vi "Add Controls in Configuration.vi"(0 "new code module":path, 1 "vi reference":refnum<vi>, 2 "configuration ctl refnum":refnum<vi>, 11 "error in":errorcluster) -> (4 "controls reference":refnum<vi>[](array[refnum]), 15 "error out":errorcluster)   [LabVIEW 2021, in "Converter.lvlib"]
uses:
  Converter.lvlib
  Converter Reusables/Converter Reusables.lvlib
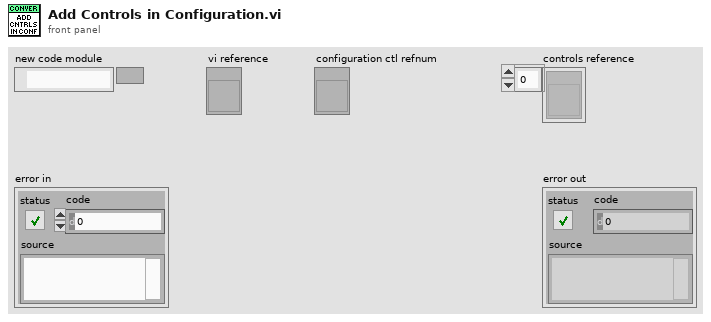
[diagram p1: front panel]
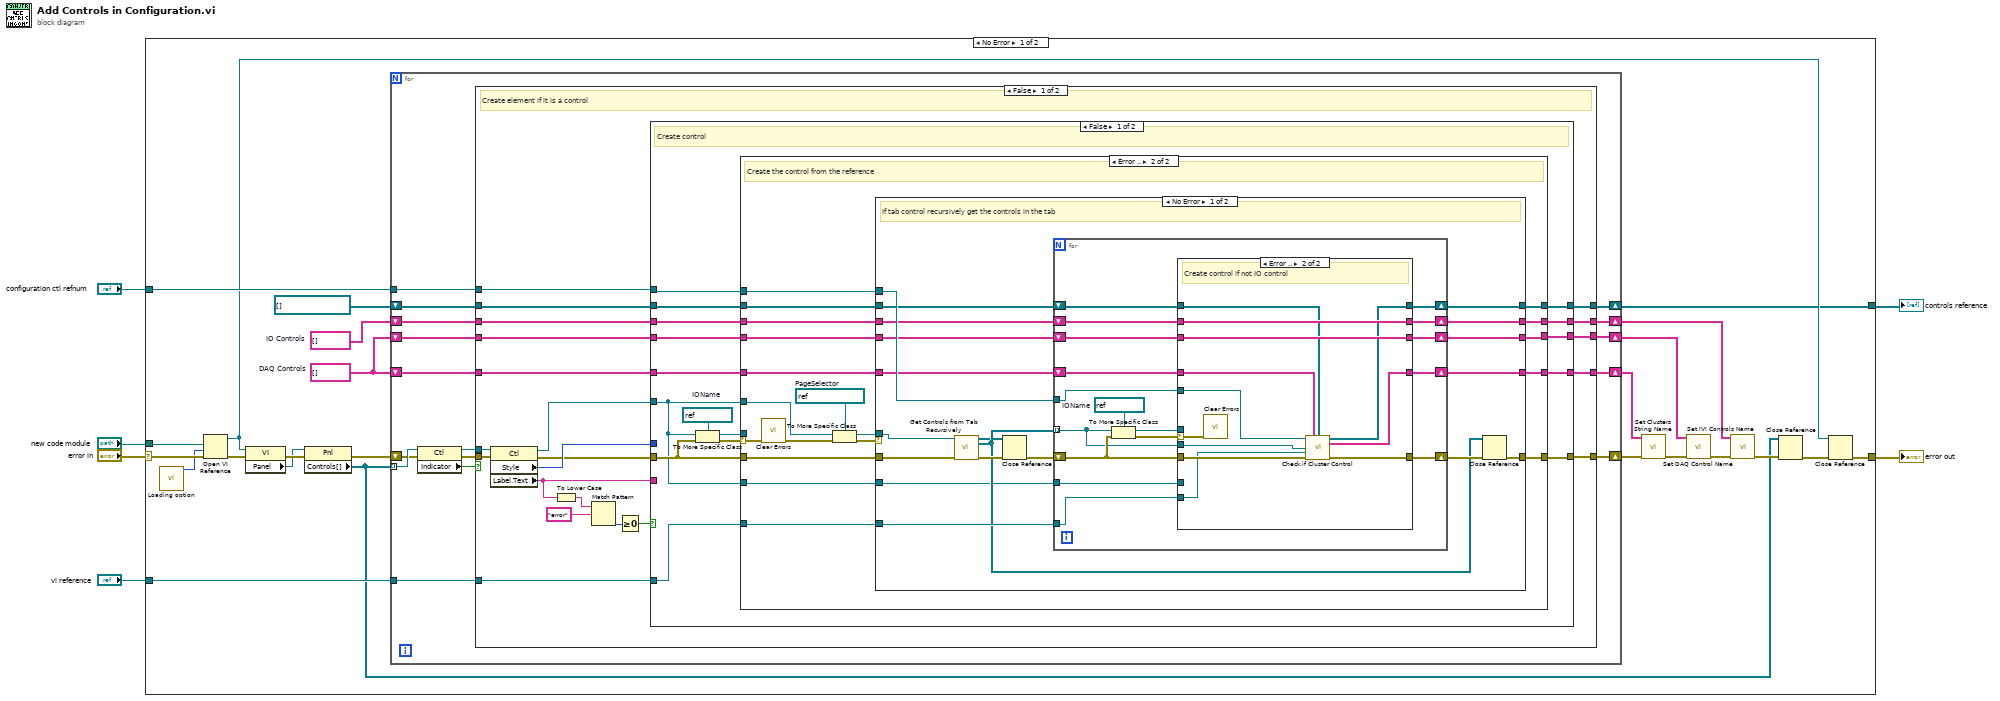
[diagram p0: block diagram]
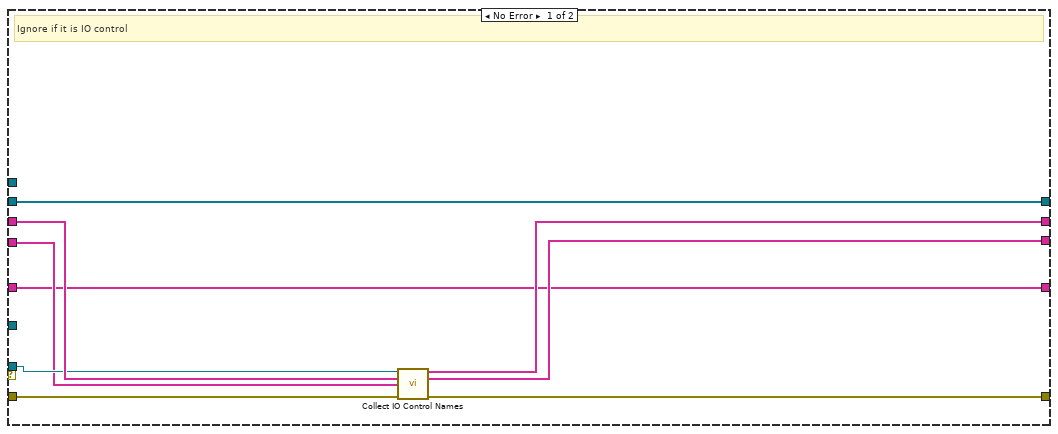
[diagram p2: hidden frame]
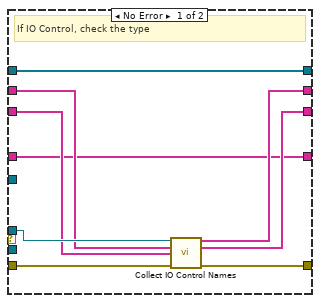
[diagram p3: hidden frame]
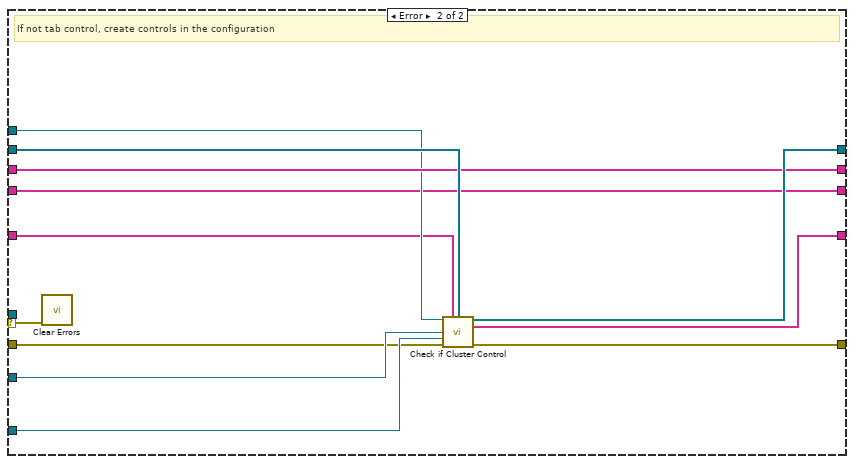
[diagram p4: hidden frame]
diagram:
  n1 = case shown="No Error" "error in" {
    selector: "error in" -> [w8 w191]
    tunnel: "configuration ctl refnum" -> [w30 _]
    tunnel: "new code module" -> [w29 _]
    tunnel: "vi reference" -> [w27 _]
    tunnel: [w25 w191] -> w3
    tunnel: [w18 _] -> w2
    frame No Error {
      w9 = string[] []  # DAQ Controls
      w16 = string[] []  # IO Controls
      n2 = call "Loading option.vi"() -> ("options"=w7:i32)  [unwired: 11 in]
      n3 = Open VI Reference(vi path=w29, options=w7, error in (no error)=w8) -> (vi reference=w22:refnum<vi>, error out=w20:errorcluster)  [unwired: 3 in]
      n4 = property class="VI"(reference=w22, error in=w20) -> (error out=w24:errorcluster, "Panel"=w23:refnum<vi>)  [unwired: 1 out]
      n5 = property class="Pnl"(reference=w23, error in=w24) -> (error out=w19:errorcluster, "Controls[]"=w21:refnum<vi>[])  [unwired: 1 out]
      n6 = for {
        tunnel: w21 -> [w44] mode=indexing
        shift-right: [w45] -> w10
        shift-left: w19 -> [w42]
        tunnel: w30 -> [w46]
        tunnel: w27 -> [w39]
        shift-right: [w38] -> w18
        shift-left: refnum<vi>[] [] -> [w37]
        shift-right: [w35] -> w17
        shift-left: w16 -> [w36]
        shift-right: [w33] -> w14
        shift-left: w9 -> [w34]
        shift-right: [w32] -> w12
        shift-left: w9 -> [w31]
        n7 = property class="Ctl"(reference=w44, error in=w42) -> (reference out=w40:refnum<vi>, error out=w41:errorcluster, "Indicator"=w43:bool)
        n8 = case shown="False" w43 {
          tunnel: w46 -> [w66 _]
          tunnel: w41 -> [w65 w190]
          tunnel: w40 -> [w64 _]
          tunnel: [w63 w190] -> w45
          tunnel: w39 -> [w56 _]
          tunnel: [w55 w189] -> w38
          tunnel: w37 -> [w54 w189]
          tunnel: w36 -> [w53 w188]
          tunnel: [w52 w188] -> w35
          tunnel: w34 -> [w51 w187]
          tunnel: [w50 w187] -> w33
          tunnel: [w49 w186] -> w32
          tunnel: w31 -> [w48 w186]
          frame False {
            # "Create element if it is a control"
            n9 = property class="Ctl"(reference=w64, error in=w65) -> (reference out=w57:refnum<vi>, error out=w47:errorcluster, "Style"=w67:u32, "Label.Text"=w62:string)
            n10 = To Lower Case(string=w62) -> (all lower case string=w58:string)
            n11 = Match Pattern(string=w58, regular expression="error") -> (offset past match=w60:i32)  [unwired: 1 in, 3 out]
            n12 = Greater Or Equal To 0?(x=w60) -> (x >= 0?=w59:bool)
            n13 = case shown="False" w59 {
              tunnel: w67 -> [_ _]
              tunnel: w66 -> [w82 _]
              tunnel: w47 -> [w83 w181]
              tunnel: w57 -> [w77 _]
              tunnel: w62 -> [_ _]
              tunnel: [w68 w181] -> w63
              tunnel: w56 -> [w81 _]
              tunnel: [w76 w185] -> w55
              tunnel: w54 -> [w75 w185]
              tunnel: w53 -> [w74 w184]
              tunnel: [w73 w184] -> w52
              tunnel: w51 -> [w72 w183]
              tunnel: [w71 w183] -> w50
              tunnel: [w70 w182] -> w49
              tunnel: w48 -> [w69 w182]
              frame False {
                w80 = refnum<vi> refnum  # IOName
                # "Create control"
                n14 = To More Specific Class(target class=w80, reference=w77, error in=w83) -> (specific class reference=w78:refnum<vi>, error out=w79:errorcluster)
                n15 = case shown="Error .." w79 {
                  selector: w79 -> [_ w108]
                  tunnel: w81 -> [_ w105]
                  tunnel: w77 -> [_ w111]
                  tunnel: w82 -> [_ w110]
                  tunnel: [w92 w109] -> w68
                  tunnel: w83 -> [w88 w107]
                  tunnel: w78 -> [w87 _]
                  tunnel: w77 -> [_ w103]
                  tunnel: [w91 w100] -> w76
                  tunnel: w75 -> [w91 w99]
                  tunnel: w74 -> [w90 w98]
                  tunnel: [w89 w97] -> w73
                  tunnel: w72 -> [w86 w96]
                  tunnel: [w85 w95] -> w71
                  tunnel: [w84 w94] -> w70
                  tunnel: w69 -> [w84 w93]
                  frame No Error {
                    # "Ignore if it is IO control"
                    n16 = call "Collect IO Control Names.vi"("io control"=w87, "io controls in"=w90, "daq controls in"=w86, "error in"=w88) -> ("io controls out"=w89:string[], "daq controls out"=w85:string[], "error out"=w92:errorcluster)  [unwired: 9 in]
                  }
                  frame Error {
                    w106 = refnum<vi> refnum  # PageSelector
                    # "Create the control from the reference"
                    n17 = call <vilib>:"Clear Errors.vi"("error in (no error)"=w108) -> ("error out"=w104:errorcluster)  [unwired: 5 in, 1 out]
                    n18 = To More Specific Class(target class=w106, reference=w103, error in=w104) -> (specific class reference=w101:refnum<vi>, error out=w102:errorcluster)
                    n19 = case shown="No Error" w102 {
                      selector: w102 -> [_ w171]
                      tunnel: w105 -> [w127 w177]
                      tunnel: w111 -> [w116 w174]
                      tunnel: w110 -> [w126 w175]
                      tunnel: [w130 w176] -> w109
                      tunnel: w107 -> [w129 w170]
                      tunnel: w101 -> [w128 _]
                      tunnel: [w114 w179] -> w100
                      tunnel: w99 -> [w115 w180]
                      tunnel: w98 -> [w125 w178]
                      tunnel: [w124 w178] -> w97
                      tunnel: w96 -> [w118 w173]
                      tunnel: [w117 w173] -> w95
                      tunnel: [w112 w169] -> w94
                      tunnel: w93 -> [w113 w172]
                      frame No Error {
                        # "If tab control recursively get the controls in the tab"
                        n20 = call "Get Controls from Tab Recursively.vi"("page sel refnum"=w128, "error in"=w129) -> ("indicators in tab"=w119:refnum<vi>[], "controls in tab"=w120:refnum<vi>[], "error out"=w122:errorcluster)  [unwired: 11 in]
                        n21 = Close Reference(reference=w119, error in (no error)=w122) -> (error out=w121:errorcluster)
                        n22 = for {
                          tunnel: w120 -> [w133] mode=indexing
                          tunnel: w127 -> [w136]
                          tunnel: w126 -> [w138]
                          shift-right: [w141] -> w124
                          shift-left: w125 -> [w145]
                          shift-right: [w142] -> w123
                          shift-left: w121 -> [w139]
                          shift-right: [w140] -> w117
                          shift-left: w118 -> [w143]
                          tunnel: w116 -> [w137]
                          shift-right: [w134] -> w114
                          shift-left: w115 -> [w135]
                          shift-right: [w131] -> w112
                          shift-left: w113 -> [w132]
                          w147 = refnum<vi> refnum  # IOName
                          n23 = To More Specific Class(target class=w147, reference=w133, error in=w139) -> (specific class reference=w146:refnum<vi>, error out=w144:errorcluster)
                          n24 = case shown="Error .." w144 {
                            selector: w144 -> [_ w166]
                            tunnel: w146 -> [w156 _]
                            tunnel: w145 -> [w155 w168]
                            tunnel: w143 -> [w154 w167]
                            tunnel: [w153 w161] -> w142
                            tunnel: [w152 w168] -> w141
                            tunnel: [w151 w167] -> w140
                            tunnel: w139 -> [w148 w162]
                            tunnel: w138 -> [_ w163]
                            tunnel: w137 -> [_ _]
                            tunnel: w136 -> [_ w159]
                            tunnel: [w150 w157] -> w134
                            tunnel: w135 -> [w150 w158]
                            tunnel: w133 -> [_ w160]
                            tunnel: w132 -> [w149 w165]
                            tunnel: [w149 w164] -> w131
                            frame No Error {
                              # "If IO Control, check the type"
                              n25 = call "Collect IO Control Names.vi"("io control"=w156, "io controls in"=w155, "daq controls in"=w154, "error in"=w148) -> ("io controls out"=w152:string[], "daq controls out"=w151:string[], "error out"=w153:errorcluster)  [unwired: 9 in]
                            }
                            frame Error {
                              # "Create control if not IO control"
                              n26 = call <vilib>:"Clear Errors.vi"("error in (no error)"=w166) -> ()  [unwired: 5 in, 2 out]
                              n27 = call "Check if Cluster Control.vi"("typedef cluster"=w163, "string controls in"=w165, "controls ref in"=w158, "ctl refnum"=w160, "vi reference"=w159, "error in"=w162) -> ("controls ref out"=w157:refnum<vi>[], "string controls out"=w164:string[], "error out"=w161:errorcluster)  [unwired: 7 in]
                            }
                          }
                        }
                        n28 = Close Reference(reference=w120, error in (no error)=w123) -> (error out=w130:errorcluster)
                      }
                      frame Error {
                        # "If not tab control, create controls in the configuration"
                        n29 = call <vilib>:"Clear Errors.vi"("error in (no error)"=w171) -> ()  [unwired: 5 in, 2 out]
                        n30 = call "Check if Cluster Control.vi"("typedef cluster"=w175, "string controls in"=w172, "controls ref in"=w180, "ctl refnum"=w174, "vi reference"=w177, "error in"=w170) -> ("controls ref out"=w179:refnum<vi>[], "string controls out"=w169:string[], "error out"=w176:errorcluster)  [unwired: 7 in]
                      }
                    }
                  }
                }
              }
              frame True {
                # "Ignore if it is error control"
              }
            }
          }
          frame True {
            # "Ignore if it is indicator"
          }
        }
      }
      n31 = call "Set Clusters String Name.vi"("controls name"=w12, "error in"=w10) -> ("error out"=w11:errorcluster)  [unwired: 13 in]
      n32 = call "Set DAQ Control Name.vi"("controls name"=w14, "error in"=w11) -> ("error out"=w13:errorcluster)  [unwired: 13 in]
      n33 = call "Set IVI Controls Name.vi"("controls name"=w17, "error in"=w13) -> ("error out"=w26:errorcluster)  [unwired: 13 in]
      n34 = Close Reference(reference=w21, error in (no error)=w26) -> (error out=w28:errorcluster)
      n35 = Close Reference(reference=w22, error in (no error)=w28) -> (error out=w25:errorcluster)
    }
    frame Error {
    }
  }
  "controls reference" <- w2
  "error out" <- w3
